vi "Extension Control.vi"(4 "Setpoint":dbl, 6 "Axis 4":dbl, 9 "Extension PID Values":cluster{"Up 1":dbl, "Down 1":dbl}={"Up 1"=2.0, "Down 1"=0.1}, 10 "Extension Setpoints":T1={"Extension Point 1"=1.2, "Extension Point 3"=1.51, "Extension Point 4"=3.5}, 11 "Feedback":dbl) -> (2 "PWM 7 Output":dbl)   [LabVIEW 2011]
uses:
  Robot Global Data.vi
panel:
  out "AI 7 Setpoint":dbl
  # "dont change here"
  # "dont change here"
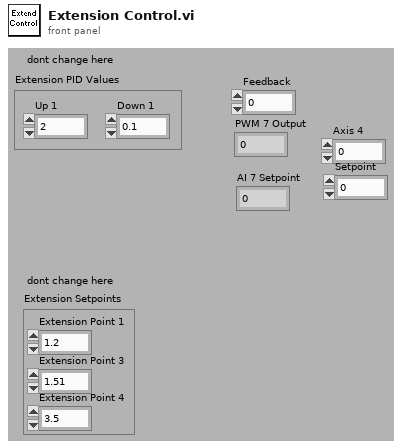
[diagram p1: front panel]
types:
  T1 = cluster{"Extension Point 1":dbl, "Extension Point 3":dbl, "Extension Point 4":dbl}
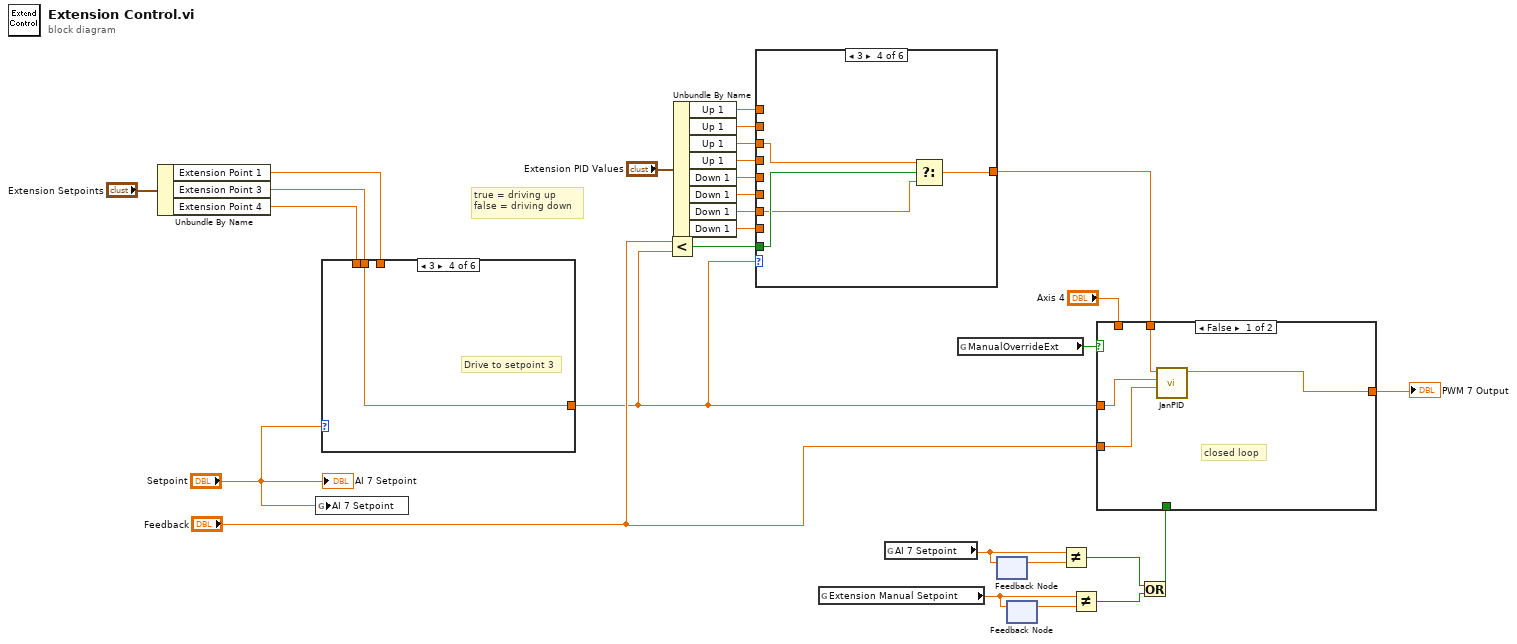
[diagram p0: block diagram]
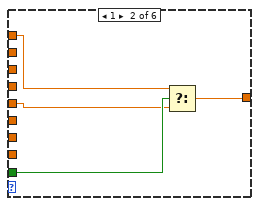
[diagram p3: hidden frame]
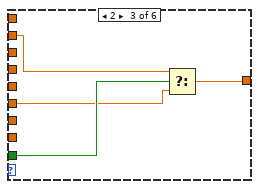
[diagram p4: hidden frame]
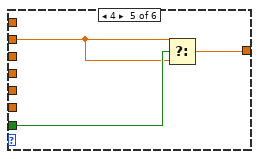
[diagram p5: hidden frame]
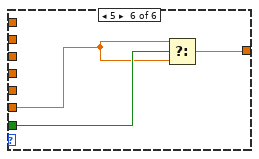
[diagram p6: hidden frame]
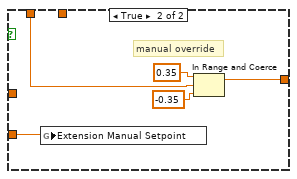
[diagram p7: hidden frame]
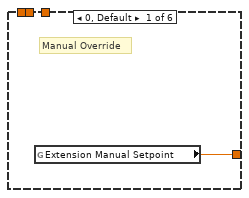
[diagram p8: hidden frame]
diagram:
  # "true = driving up\nfalse = driving down"
  n1 = Unbundle By Name("Extension Setpoints") -> ("Extension Point 1"=w27:dbl, "Extension Point 3"=w26:dbl, "Extension Point 4"=w25:dbl)
  n2 = global write "Robot Global Data.vi" "AI 7 Setpoint"("Setpoint") -> ()
  n3 = case shown="3" "Setpoint" {
    tunnel: [w29 w30 w31 w32 w33 w34] -> w1
    tunnel: w27 -> [_ w30 w31 _ _ w34]
    tunnel: w26 -> [_ _ _ w32 _ _]
    tunnel: w25 -> [_ _ _ _ w33 _]
    frame 0, Default {
      # "Manual Override"
      n4 = global read "Robot Global Data.vi" "Extension Manual Setpoint"() -> (w29:dbl)
    }
    frame 1 {
      # "Drive to setpoint 1"
    }
    frame 2 {
      # "Drive to setpoint 2"
    }
    frame 3 {
      # "Drive to setpoint 3"
    }
    frame 4 {
      # "Drive to setpoint 4"
    }
    frame 5 {
      # "neutral (tube carry)"
    }
  }
  n5 = Less?(x="Feedback", y=w1) -> (x < y?=w14:bool)
  n6 = Unbundle By Name("Extension PID Values") -> ("Up 1"=w23:dbl, "Up 1"=w22:dbl, "Up 1"=w21:dbl, "Up 1"=w20:dbl, "Down 1"=w19:dbl, "Down 1"=w18:dbl, "Down 1"=w17:dbl, "Down 1"=w16:dbl)
  n7 = case shown="3" w1 {
    tunnel: w23 -> [w35 w37 _ _ _ _]
    tunnel: w22 -> [_ _ w41 _ _ _]
    tunnel: w21 -> [_ _ _ w45 _ _]
    tunnel: w20 -> [_ _ _ _ w48 _]
    tunnel: w19 -> [_ w36 _ _ _ _]
    tunnel: w18 -> [_ _ w40 _ _ _]
    tunnel: w17 -> [_ _ _ w44 _ _]
    tunnel: w16 -> [_ _ _ _ _ w51]
    tunnel: w14 -> [_ w39 w43 w47 w50 w53]
    tunnel: [w35 w38 w42 w46 w49 w52] -> w13
    frame 0, Default {
    }
    frame 1 {
      n8 = Select(t=w37, s=w39, f=w36) -> (s? t:f=w38:dbl)
    }
    frame 2 {
      n9 = Select(t=w41, s=w43, f=w40) -> (s? t:f=w42:dbl)
    }
    frame 3 {
      n10 = Select(t=w45, s=w47, f=w44) -> (s? t:f=w46:dbl)
    }
    frame 4 {
      n11 = Select(t=w48, s=w50, f=w48) -> (s? t:f=w49:dbl)
    }
    frame 5 {
      n12 = Select(t=w51, s=w53, f=w51) -> (s? t:f=w52:dbl)
    }
  }
  n13 = global read "Robot Global Data.vi" "Extension Manual Setpoint"() -> (w8:dbl)
  n14 = global read "Robot Global Data.vi" "AI 7 Setpoint"() -> (w11:dbl)
  n15 = global read "Robot Global Data.vi" "ManualOverrideExt"() -> (w2:bool)
  n16 = feedback-in #1(w11) -> ()
  n17 = feedback #1() -> (w10:dbl)  [unwired: 1 out]
  n18 = feedback-in #2(w8) -> ()
  n19 = feedback #2() -> (w9:dbl)  [unwired: 1 out]
  n20 = Not Equal?(x=w11, y=w10) -> (x != y?=w6:bool)
  n21 = Not Equal?(x=w8, y=w9) -> (x != y?=w7:bool)
  n22 = Or(x=w6, y=w7) -> (x .or. y?=w5:bool)
  n23 = case shown="False" w2 {
    tunnel: [w57 w58] -> w15
    tunnel: "Feedback" -> [w54 w62]
    tunnel: w1 -> [w55 _]
    tunnel: w13 -> [w56 _]
    tunnel: "Axis 4" -> [_ w59]
    tunnel: w5 -> [_ _]
    frame False {
      # "closed loop"
      n24 = call "JanPID.vi"("Feedback"=w54, "Setpoint"=w55, "P"=w56) -> ("Motor Output"=w57:dbl)  [unwired: 1 in, 7 out]
    }
    frame True {
      # "manual override"
      n25 = global write "Robot Global Data.vi" "Extension Manual Setpoint"(w62) -> ()
      n26 = In Range and Coerce(upper limit=0.35, x=w59, lower limit=-0.35) -> (coerced(x)=w58:dbl)  [unwired: 1 out]
    }
  }
  "PWM 7 Output" <- w15
  "AI 7 Setpoint" <- "Setpoint"
